vi "Util_Convert_from_m.vi"(2 "distance (m) wheel":dbl) -> (0 "rotations gear":dbl)   [LabVIEW 2009, in "OWNCAN.lvlib"]
uses:
  OWNCAN.lvlib
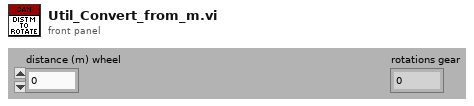
[diagram p1: front panel]
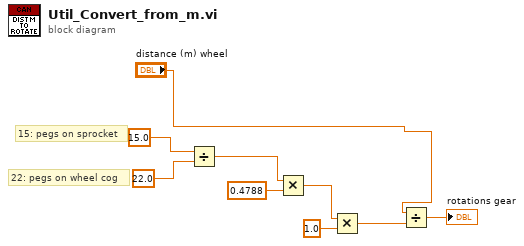
[diagram p0: block diagram]
diagram:
  # "22: pegs on wheel cog"
  # "15: pegs on sprocket"
  n1 = Divide(x=15.0, y=22.0) -> (x/y=w7:dbl)
  n2 = Multiply(x=w7, y=0.4788) -> (x*y=w5:dbl)
  n3 = Multiply(x=w5, y=1.0) -> (x*y=w3:dbl)
  n4 = Divide(x="distance (m) wheel", y=w3) -> (x/y=→"rotations gear":dbl)
